vi "GetImage From ClipBoard.vi"(8 "错误输入（无错误）":errorcluster, 11 "Image Depth":i32) -> (0 "错误输出":errorcluster, 3 "new picture":picture caption="新图片")   [LabVIEW 2012, in "Application.lvlib"]
uses:
  Application.lvlib
  <vilib>/picture/picture.llb/imagedata.ctl
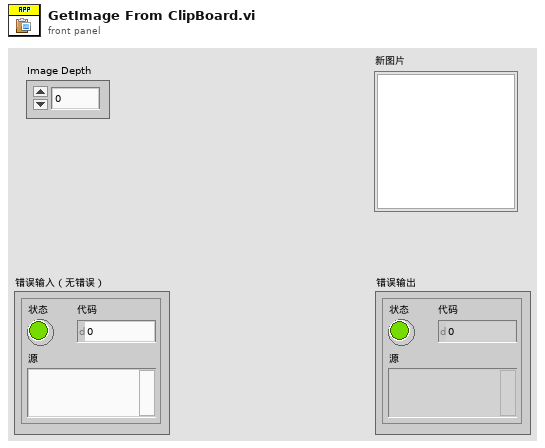
[diagram p1: front panel]
types:
  T1 = typedef "imagedata.ctl" = cluster{"image type":i32, "image depth":i32, "image":u8[], "mask":u8[], "colors":u32[], "Rectangle":cluster{"left":i16, "top":i16, "right":i16, "bottom":i16}}
  T2 = typedef "LVRectTypeDef.ctl" = cluster{"left":i16, "top":i16, "right":i16, "bottom":i16}
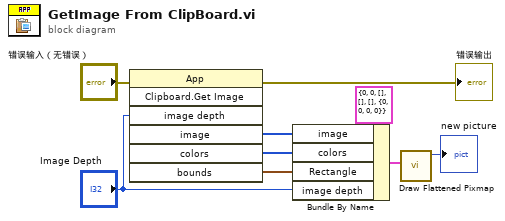
[diagram p0: block diagram]
diagram:
  n1 = invoke class="App" method="Clipboard.Get Image"(error in="错误输入（无错误）", "image depth"="Image Depth") -> (error out=→"错误输出":errorcluster, "image"=w8:u8[], "colors"=w7:u32[], "bounds"=w6:T2)  [unwired: 5 in, 3 out]
  n2 = Bundle By Name(cluster=T1 {"image type"=0, "image depth"=0, "image"=[], "mask"=[], "colors"=[], "Rectangle"={"left"=0, "top"=0, "right"=0, "bottom"=0}} ("image data"), "image"=w8, "colors"=w7, "Rectangle"=w6, "image depth"="Image Depth") -> (w5:T1)
  n3 = call <vilib>:"Draw Flattened Pixmap.vi"("image data"=w5) -> ("new picture"=→"new picture":picture)  [unwired: 8 in]
